vi "DTMF Packet Receiver.vi"() -> ()   [LabVIEW 2011]
uses:
  subVIs_USRP/sub_Chop_Packet.vi
  subVIs_USRP/sub_Ave_Power_And_Thresholding.vi
  subVIs_USRP/sub_Extract_Packet_Boundaries - G.vi
  subVIs_USRP/sub_Extract_Packets.vi
  <instrlib>/niUSRP/niUSRP Fetch Rx Data (CDB Cluster).vi
  subVIs_USRP/subDCOffset.vi
  subVIs_USRP/sub_est_noise_power - G1.vi
  subVIs_DTMF_Student/Proj3_Wireless_DTMF_Receiver.vi
  <vilib>/addons/Modulation/niDMT.lvlib
panel:
  in  "threshold":dbl=97.0
  out "Constellation Graph":T1(graph)
  out "Symbol Rate\n[symbols/sec]":dbl=25000.0 format="%#.6p"
  in  "synchronization parameters":T2={"expected sync location (symbols)"=-1, "sync sequence"=[], "sync location uncertainty (symbols)"=0, "sync indent (symbols)"=0} {"sync sequence" format="%.2f"}
  in  "stop":bool
  in  "Tab Control":T3(tab)=enum."Rx Parameters"
  in  "PN Sequence Order for Sync":i32=31
  in  "Packet Parameters":T4={"Guard Bits "=30, "Sync Bits"=20, "Message Bits"=1024, "Number of Packets \nto Expect"=47}
  out "Received Signal (Raw)":dbl[](graph)
  out "Successfully Received Pkt Num":bool[][](array[boolean])
  out "Packet Reception Percentage (%)":dbl(slide) scale=0.0..100.0
  out "Received Quantized DTMF Signal":dbl[](graph)
  in  "DTMF Settings":T5={"My Phone Number"="", "Ring Tone"=FALSE, "Quantization Level"=4, "\nGray Encoding"=FALSE} {"Quantization Level" items=["2"=2, "4"=4, "8"=8, "16"=16]}
  out "Recovered Message":string
  out "Successfully Received Pkt Num.":bool[][](array[boolean])
  out "Received Digits":string
  in  "Ringtone Path":path=path "C:/Users/Sungeun/Dropbox/Lab/DTMF/VI Source/Project 3/ringtone/Nokia_Original.wav"
  in  "Choose a PSK Format":T6(tab)=enum."QPSK" caption="PSK"
  in  "BPSK System Parameters":T7={"Samples per Symbol"=8, "symbol map"=[], "Differential PSK"=enum."disable", "PSK type"=0} {"PSK type" items=["normal", "shifted", "offset"]; "symbol map" format="%.3f"}
  in  "QPSK System Parameters":T7={"Samples per Symbol"=8, "symbol map"=[], "Differential PSK"=enum."disable", "PSK type"=0} {"PSK type" items=["normal", "shifted", "offset"]; "symbol map" format="%.3f"}
  in  "pi/4 DQPSK System Parameters":T7={"Samples per Symbol"=8, "symbol map"=[], "Differential PSK"=enum."enable", "PSK type"=1} {"PSK type" items=["normal", "shifted", "offset"]; "symbol map" format="%.3f"}
  in  "OQPSK System Parameters":T7={"Samples per Symbol"=8, "symbol map"=[], "Differential PSK"=enum."disable", "PSK type"=2} {"PSK type" items=["normal", "shifted", "offset"]; "symbol map" format="%.3f"}
  in  "8-PSK System Parameters":T7={"Samples per Symbol"=8, "symbol map"=[], "Differential PSK"=enum."disable", "PSK type"=0} {"PSK type" items=["normal", "shifted", "offset"]; "symbol map" format="%.3f"}
  in  "16-PSK System Parameters":T7={"Samples per Symbol"=8, "symbol map"=[], "Differential PSK"=enum."disable", "PSK type"=0} {"PSK type" items=["normal", "shifted", "offset"]; "symbol map" format="%.3f"}
  in  "M":i32=4 min=2 step=2
  in  "Custom System Parameters":T7={"Samples per Symbol"=8, "symbol map"=[], "Differential PSK"=enum."disable", "PSK type"=0} {"PSK type" items=["normal", "shifted", "offset"]; "symbol map" format="%.3f"}
  in  "filter parameters":T8={"Alpha"=0.5, "Filter Length"=6, "TX Filter"=enum."Root Raised Cos"} caption="Matching Filter Parameters" {"Alpha" format="%.2f"}
  in  "Acquisition Duration [sec]":dbl=0.06 format="%#.6p"
  in  "Rx Parameters":T9={"Rx IQ Sampling\nRate [s/sec]"=200000.0, "Rx\nFrequency [Hz]"=915000000.0, "Rx Gain [dB]"=20.0, "Rx Antenna"="RX1"} {"Rx Gain [dB]" format="%#.6p"; "Rx\nFrequency [Hz]" format="%#.6p"; "Rx IQ Sampling\nRate [s/sec]" format="%#.6p"}
  out "Actual Rx Parameters":T9={"Rx IQ Sampling\nRate [s/sec]"=200000.0, "Rx\nFrequency [Hz]"=2500000000.0, "Rx Gain [dB]"=20.0, "Rx Antenna"="RX1"} {"Rx Gain [dB]" format="%#.6p"; "Rx\nFrequency [Hz]" format="%#.6p"; "Rx IQ Sampling\nRate [s/sec]" format="%#.6p"}
  in  "USRP IP Address":refnum<k15>="192.168.10.3"
  out "SNR [dB]":dbl
  out "Sync Found":bool=TRUE
  out "Correct Packets Rx":i16=46
  in  "Continuous Acquire?":bool
  out "Singal & Noise Power":cluster{"signal_power":dbl, "noise_power":dbl}={"signal_power"=0.001168884890875219, "noise_power"=5.163954192250838e-08}
  out "error out":errorcluster
  out "Cumulative Packets Recovered":i16(graph)
  out "Signal and Noise Power Tracking":cluster{"total_power":dbl, "noise_power":dbl}(graph)={"total_power"=0.001168884890875219, "noise_power"=5.163954192250838e-08}
  # "DTMF Packet Receiver"
  # "Guard\nBand"
  # "Sync\nSeq"
  # "Packet\nNumber"
  # "Pad\nData"
  # "Blank\nFrame"
  # "Data"
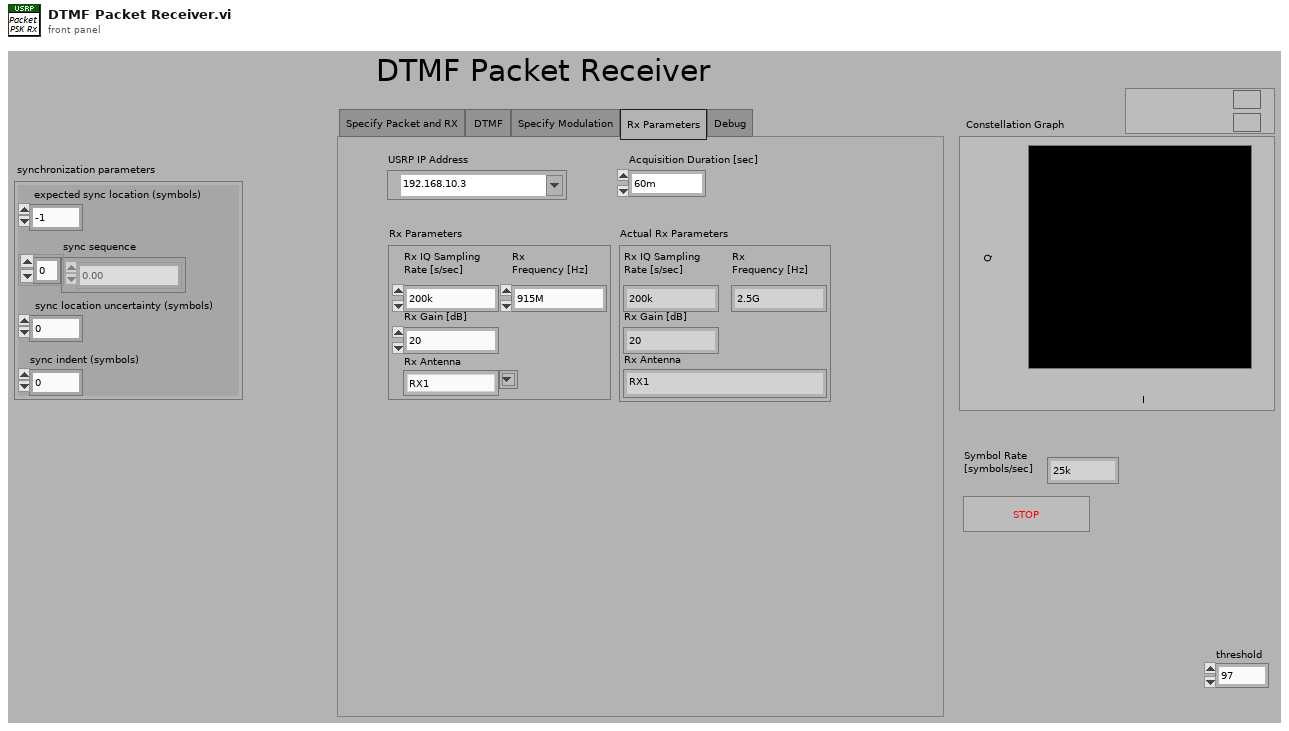
[diagram p1: front panel]
types:
  T1 = cluster{"Decimated Array":dbl[], "Decimated Array":dbl[]}[]
  T2 = cluster{"expected sync location (symbols)":i32, "sync sequence":cdb[], "sync location uncertainty (symbols)":i32, "sync indent (symbols)":i32}
  T3 = enum32{"Specify Packet and RX", "DTMF ", "Specify Modulation", "Rx Parameters", "Debug"}
  T4 = cluster{"Guard Bits ":i32, "Sync Bits":i32, "Message Bits":i32, "Number of Packets \nto Expect":i32}
  T5 = cluster{"My Phone Number":string, "Ring Tone":bool, "Quantization Level":u16, "\nGray Encoding":bool}
  T6 = enum32{"BPSK", "QPSK", "pi/4DQPSK", "OQPSK", "8-PSK", "16-PSK", "Custom"}
  T7 = cluster{"Samples per Symbol":i32, "symbol map":cdb[], "Differential PSK":enum16{"disable", "enable"}, "PSK type":u16}
  T8 = cluster{"Alpha":dbl, "Filter Length":i32, "TX Filter":enum16{"none", "Raised Cosine", "Root Raised Cos", "Gaussian"}}
  T9 = cluster{"Rx IQ Sampling\nRate [s/sec]":dbl, "Rx\nFrequency [Hz]":dbl, "Rx Gain [dB]":dbl, "Rx Antenna":string}
  T10 = cluster{"Packet Array":i32[][], "IP Array of Pkt Nums Received  ":bool[]}
  T11 = cluster{"bit stream ":i8[][], "Sync Valid?":bool[], "Decoded Pkt Numbers":u32[], "Enable?":bool}
  T12 = cluster{"packet_arr":cdb[][], "Packets Valid?":bool}
  T13 = cluster{"PSK type":u16, "Samples per Symbol":i32, "Differential PSK":enum16{"disable", "enable"}, "M":i32}
  T14 = cluster{"PSK system parameters":cluster{"samples per symbol (16)":i32, "symbol map":cdb[], "differential PSK":enum16{"disable", "enable"}, "PSK type":u16}, "pulse shaping filter coefficients":dbl[], "matched filter coefficients":dbl[], "synchronization parameters":cluster{"expected sync location (symbols)":i32, "sync sequence":cdb[], "sync location uncertainty (symbols)":i32, "sync indent (symbols)":i32}, "Sync Bits":i8[]}
  T15 = typedef "niAMT.lvlib/Complex Data Waveform.ctl" = cluster{"t0":dbl, "dt":dbl, "Y":cdb[]}
  T16 = cluster{"constellation":dbl[], "oversampled data":dbl[]}[]
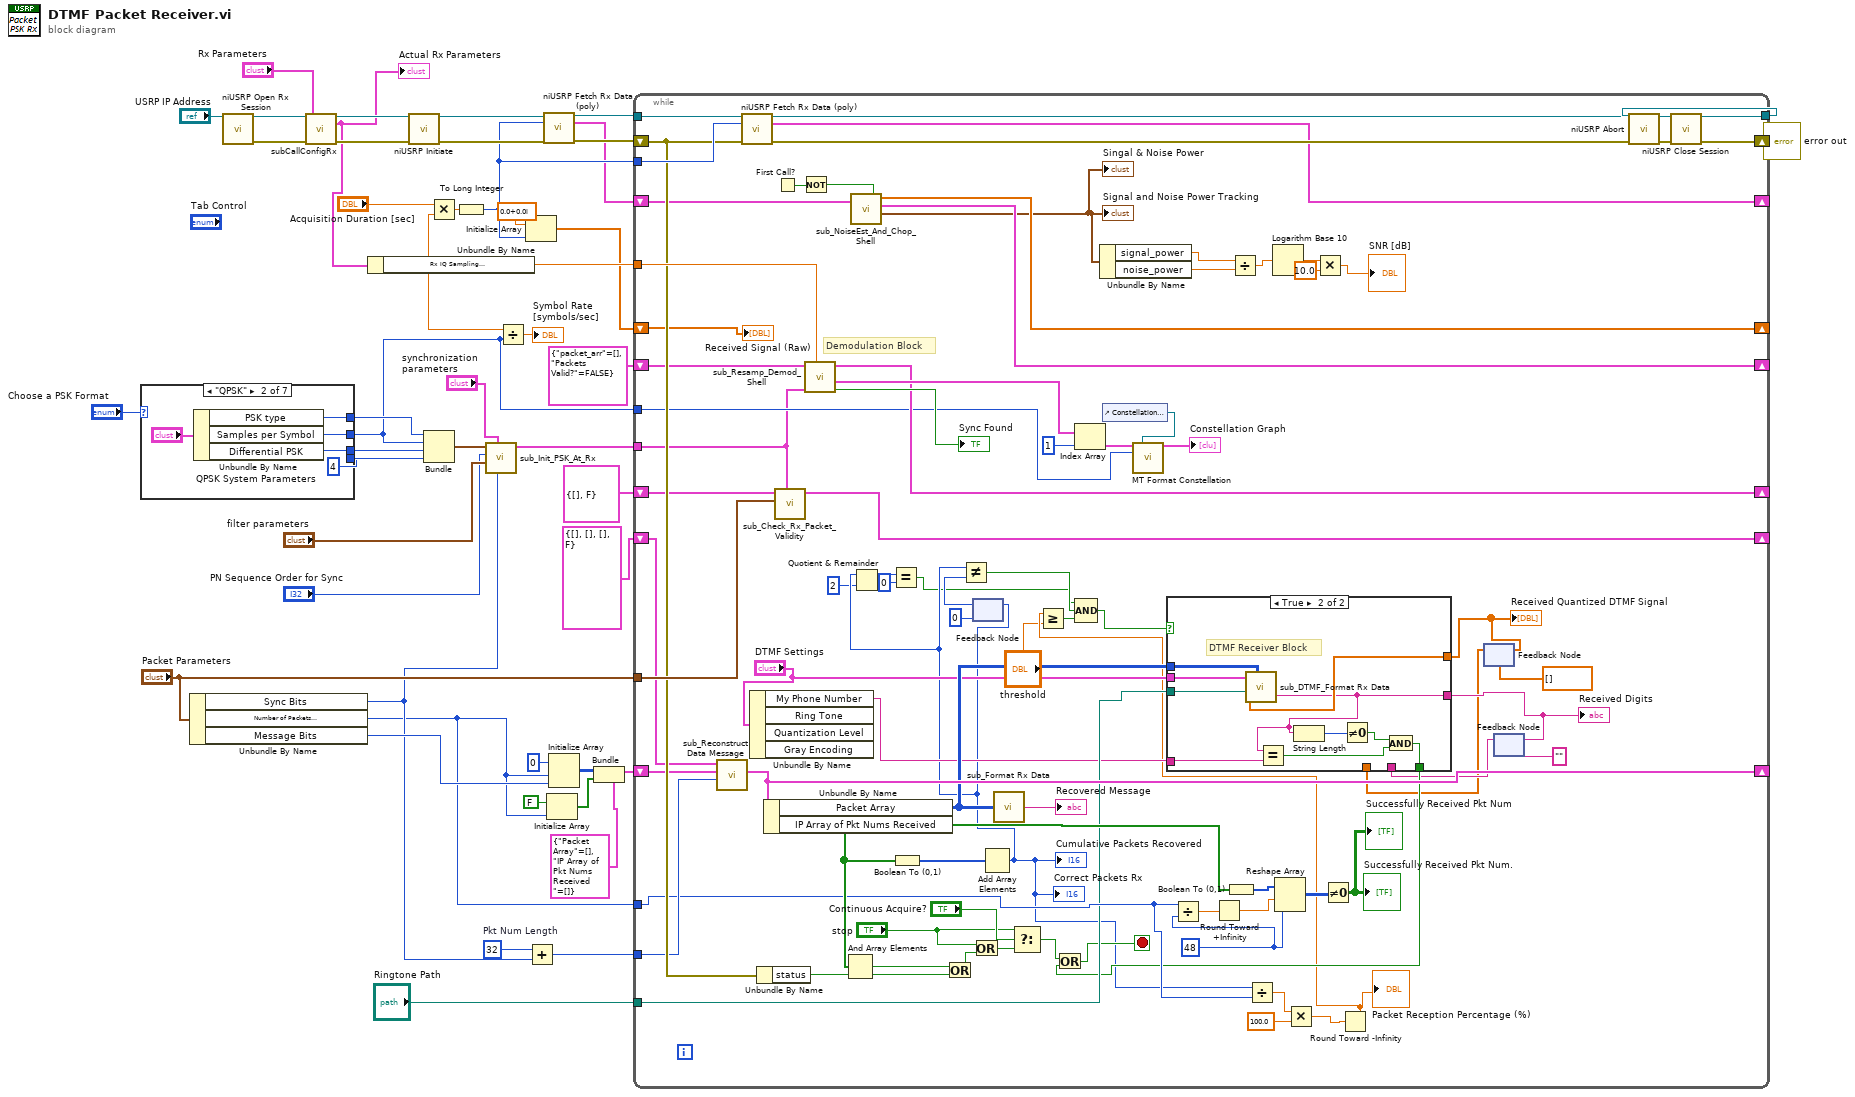
[diagram p0: block diagram]
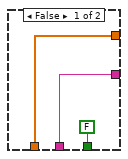
[diagram p2: hidden frame]
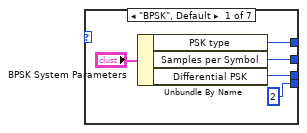
[diagram p3: hidden frame]
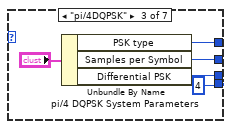
[diagram p4: hidden frame]
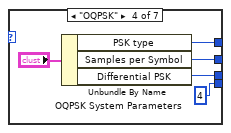
[diagram p5: hidden frame]
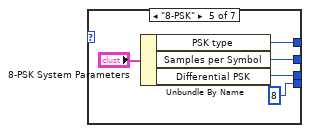
[diagram p6: hidden frame]
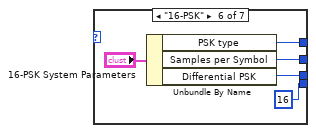
[diagram p7: hidden frame]
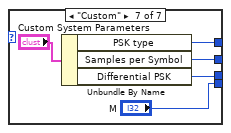
[diagram p8: hidden frame]
diagram:
  w26 = 32  # Pkt Num Length
  n1 = case shown="\"QPSK\"" "Choose a PSK Format" {
    tunnel: [w53 w59 w64 w69 w74 w80 w83] -> w24
    tunnel: [w54 w57 w63 w68 w73 w79 w84] -> w34
    tunnel: [2 ("M-PSK (4)") 4 ("M-PSK (4)") 4 ("M-PSK (4)") 4 ("M-PSK (4)") 8 ("M-PSK (4)") 16 ("M-PSK (4)") "M"] -> w33
    tunnel: [w55 w58 w62 w67 w75 w78 w85] -> w35
    frame "BPSK", Default {
      n2 = Unbundle By Name("BPSK System Parameters") -> ("PSK type"=w55:u16, "Samples per Symbol"=w53:i32, "Differential PSK"=w54:enum16{"disable", "enable"})
    }
    frame "QPSK" {
      n3 = Unbundle By Name("QPSK System Parameters") -> ("PSK type"=w58:u16, "Samples per Symbol"=w59:i32, "Differential PSK"=w57:enum16{"disable", "enable"})
    }
    frame "pi/4DQPSK" {
      n4 = Unbundle By Name("pi/4 DQPSK System Parameters") -> ("PSK type"=w62:u16, "Samples per Symbol"=w64:i32, "Differential PSK"=w63:enum16{"disable", "enable"})
    }
    frame "OQPSK" {
      n5 = Unbundle By Name("OQPSK System Parameters") -> ("PSK type"=w67:u16, "Samples per Symbol"=w69:i32, "Differential PSK"=w68:enum16{"disable", "enable"})
    }
    frame "8-PSK" {
      n6 = Unbundle By Name("8-PSK System Parameters") -> ("PSK type"=w75:u16, "Samples per Symbol"=w74:i32, "Differential PSK"=w73:enum16{"disable", "enable"})
    }
    frame "16-PSK" {
      n7 = Unbundle By Name("16-PSK System Parameters") -> ("PSK type"=w78:u16, "Samples per Symbol"=w80:i32, "Differential PSK"=w79:enum16{"disable", "enable"})
    }
    frame "Custom" {
      n8 = Unbundle By Name("Custom System Parameters") -> ("PSK type"=w85:u16, "Samples per Symbol"=w83:i32, "Differential PSK"=w84:enum16{"disable", "enable"})
    }
  }
  n9 = Unbundle By Name("Packet Parameters") -> ("Sync Bits"=w10:i32, "Number of Packets \nto Expect"=w2:i32, "Message Bits"=w25:i32)
  n10 = call <instrlib>:"niUSRP Open Rx Session.vi"("device names"="USRP IP Address") -> ("session handle out"=w46:refnum<k15>, "error out"=w47:errorcluster)  [unwired: 13 in]
  n11 = call "subCallConfigRx.vi"("session handle"=w46, "Rx Parameters"="Rx Parameters", "error in"=w47) -> ("session handle out"=w44:refnum<k15>, "Actual Rx Parameters"=w27:T9, "error out"=w43:errorcluster)  [unwired: 10 in]
  "Actual Rx Parameters" <- w27
  n12 = Unbundle By Name(w27) -> ("Rx IQ Sampling\nRate [s/sec]"=w21:dbl)
  n13 = call <instrlib>:"niUSRP Initiate.vi"("session handle"=w44, "error in (no error)"=w43) -> ("session handle out"=w6:refnum<k15>, "error out"=w5:errorcluster)  [unwired: 12 in]
  n14 = Bundle("PSK type"=w35, "Samples per Symbol"=w24, "Differential PSK"=w34, "M"=w33) -> (w31:T13)  [unwired: 1 in]
  n15 = Multiply(x="Acquisition Duration [sec]", y=w21) -> (x*y=w49:dbl)
  n16 = To Long Integer(number=w49) -> (32bit integer=w4:i32)
  n17 = call "sub_Init_PSK_At_Rx.vi"("Sync Bits"=w10, "synchronization parameters"="synchronization parameters", "filter parameters"="filter parameters", "PN sequence order (9)"="PN Sequence Order for Sync", "PSK Parameters"=w31) -> ("PSK Init Parameters"=w30:T14)  [unwired: 5 in, 1 out]
  n18 = Divide(x=w21, y=w24) -> (x/y=→"Symbol Rate\n[symbols/sec]":dbl)
  n19 = Initialize Array(cdb 0.0+0.0i ("element"), w4) -> (w12:cdb[])
  n20 = Add(x=w26, y=w10) -> (x+y=w36:i32)
  n21 = call-poly <instrlib>:"niUSRP Fetch Rx Data (poly).vi"("session handle"=w6, "number of samples"=w4, "error in (no error)"=w5) -> ("session handle out"=w8:refnum<k15>, "data"=w3:cluster{"t0":dbl, "dt":dbl, "Y":cdb[]}, "error out"=w7:errorcluster)  [unwired: 9 in, 1 out]
  n22 = Initialize Array(FALSE, w2) -> (w14:bool[])
  n23 = Initialize Array(0, w2, w25) -> (w15:i32[][])
  n24 = Bundle(cluster=T10 {"Packet Array"=[], "IP Array of Pkt Nums Received  "=[]} ("Packet Info"), "Packet Array"=w15, "IP Array of Pkt Nums Received"=w14) -> (w13:T10)
  n25 = while {
    tunnel: w21 -> [w166]
    tunnel: w8 -> [w151]
    tunnel: [w149] -> w40
    tunnel: w4 -> [w148]
    tunnel: "Packet Parameters" -> [w165]
    tunnel: w36 -> [w135]
    tunnel: w30 -> [w131]
    shift-right: [w150] -> w39
    shift-left: w7 -> [w146]
    tunnel: w24 -> [w132]
    shift-right: [w134] -> _
    shift-left: w13 -> [w136]
    shift-right: [w142] -> _
    shift-left: T12 {"packet_arr"=[], "Packets Valid?"=FALSE} -> [w143]
    shift-right: [w138] -> _
    shift-left: cluster{"bit stream":i8[][], "Enable?":bool} {"bit stream"=[], "Enable?"=FALSE} ("Output Bitstream") -> [w141]
    shift-right: [w130] -> _
    shift-left: T11 {"bit stream "=[], "Sync Valid?"=[], "Decoded Pkt Numbers"=[], "Enable?"=FALSE} ("Output Bit Stream") -> [w137]
    shift-right: [w139] -> _
    shift-left: w3 -> [w140]
    shift-right: [w133] -> _
    shift-left: w12 -> [w120]
    tunnel: w2 -> [w121]
    tunnel: "Ringtone Path" -> [w108]
    stop <- w104 stop-if-true
    w124 = 48 ("dimension size")
    # "Demodulation Block"
    n26 = call "sub_Reconstruct Data Message.vi"("Start Loc of Data"=w135, "Packet Info"=w136, "Input Stream"=w137) -> ("Packet Info out"=w134:T10)  [unwired: 8 in]
    n27 = call-poly <instrlib>:"niUSRP Fetch Rx Data (poly).vi"("session handle"=w151, "number of samples"=w148, "error in (no error)"=w146) -> ("session handle out"=w149:refnum<k15>, "data"=w139:cluster{"t0":dbl, "dt":dbl, "Y":cdb[]}, "error out"=w150:errorcluster)  [unwired: 9 in, 1 out]
    n28 = Unbundle By Name("DTMF Settings") -> ("My Phone Number"=w107:string)  [unwired: 3 out]
    n29 = Unbundle By Name(w146) -> ("status"=w145:bool)
    n30 = Unbundle By Name(w134) -> ("Packet Array"=w129:i32[][], "IP Array of Pkt Nums Received"=w128:bool[])
    n31 = First Call?() -> (First Call?: T/F=w153:bool)
    n32 = call "sub_Check_Rx_Packet_Validity.vi"("PSK Init Parameters"=w131, "Packet Parameters"=w165, "Input Bit Stream"=w141) -> ("Output Bit Stream"=w130:T11)  [unwired: 7 in]
    n33 = Not(x=w153) -> (.not. x?=w152:bool)
    n34 = call "sub_Resamp_Demod_Shell.vi"("Rx IQ Sampling\nRate [s/sec]"=w166, "PSK Init Parameters"=w131, "Input Packets"=w143) -> ("Synch Found?"=→"Sync Found":bool, "recovered complex waveform"=w156:T15[], "Output Bitstream"=w138:cluster{"bit stream":i8[][], "Enable?":bool})  [unwired: 3 in]
    n35 = And Array Elements(Boolean array=w128) -> (logical AND=w147:bool)
    n36 = call "sub_NoiseEst_And_Chop_Shell.vi"("data"=w140, "Enable"=w152) -> ("Singal & Noise Power"=w115:cluster{"signal_power":dbl, "noise_power":dbl}, "Output Packets"=w142:cluster{"Packets":cdb[][], "Enable?":bool}, "Delay signal (for plotting use only)"=w133:cdb[])  [unwired: 3 in]
    "Signal and Noise Power Tracking" <- w115
    "Singal & Noise Power" <- w115
    n37 = Boolean To (0,1)(Boolean=w128) -> (0, 1=w164:i16[])
    n38 = Or(x=w147, y=w145) -> (x .or. y?=w144:bool)
    n39 = Or(x="stop", y=w144) -> (x .or. y?=w162:bool)
    n40 = feedback #1(i16 0) -> (w98:i16)
    n41 = Add Array Elements(numeric array=w164) -> (sum=w88:i16)
    "Correct Packets Rx" <- w88
    "Cumulative Packets Recovered" <- w88
    n42 = Quotient & Remainder(x=w88, y=i16 2) -> (x-y*floor(x/y)=w90:i16)  [unwired: 1 out]
    n43 = Equal?(x=w90, y=i16 0) -> (x = y?=w86:bool)
    n44 = Not Equal?(x=w88, y=w98) -> (x != y?=w97:bool)
    n45 = feedback-in #1(w88) -> ()
    n46 = call "sub_Format Rx Data.vi"("Output Packet Array"=w129) -> ("Received Message"=→"Recovered Message":string)
    n47 = Select(t="stop", s="Continuous Acquire?", f=w162) -> (s? t:f=w106:bool)
    n48 = Index Array(array=w156, index=1) -> (element=w155:T15)
    n49 = Unbundle By Name(w115) -> ("signal_power"=w114:dbl, "noise_power"=w113:dbl)
    n50 = control-ref of="Constellation Graph"() -> (w158:refnum<vi>)
    n51 = call <vilib>:"MT Format Constellation.vi"("waveform"=w155, "constellation reference"=w158, "samples per symbol"=w132) -> ("constellation graph"=→"Constellation Graph":T16)  [unwired: 2 in, 10 out]
    n52 = Divide(x=w121, y=w124) -> (x/y=w123:dbl)
    n53 = Round Toward +Infinity(x=w123) -> (ceil(x): smallest int >= x=w122:dbl)
    n54 = Boolean To (0,1)(Boolean=w128) -> (0, 1=w127:i16[])
    n55 = Divide(x=w114, y=w113) -> (x/y=w112:dbl)
    n56 = Divide(x=w88, y=w121) -> (x/y=w117:dbl)
    n57 = Logarithm Base 10(1:w112) -> (0:w111:dbl)
    n58 = Reshape Array(w127, w122, w124) -> (w126:i16[][])
    n59 = Multiply(x=w117, y=100.0) -> (x*y=w116:dbl)
    n60 = Multiply(x=w111, y=10.0) -> (x*y=→"SNR [dB]":dbl)
    n61 = Not Equal To 0?(x=w126) -> (x != 0?=→"Successfully Received Pkt Num." →"Successfully Received Pkt Num":bool[][])
    n62 = Round Toward -Infinity(1:w116) -> (0:w103:dbl)
    "Packet Reception Percentage (%)" <- w103
    n63 = Greater Or Equal?(x=w103, y="threshold") -> (x >= y?=w101:bool)
    n64 = Compound Arithmetic op=AND(w86, w97, w101) -> (w100:bool)
    n65 = feedback #2(dbl[] [] ("dequants")) -> (w93:dbl[])
    n66 = feedback #3("" ("Received Digits")) -> (w95:string)
    n67 = case shown="True" w100 {
      tunnel: w129 -> [_ w179]
      tunnel: "DTMF Settings" -> [_ w178]
      tunnel: [w167 w177] -> w94
      tunnel: w108 -> [_ w176]
      tunnel: [w168 w172] -> w96
      tunnel: w107 -> [_ w171]
      tunnel: [FALSE w170] -> w105
      tunnel: w95 -> [w168 _]
      tunnel: w93 -> [w167 _]
      frame False {
      }
      frame True {
        # "DTMF Receiver Block"
        n68 = call "sub_DTMF_Format Rx Data.vi"("DTMF Settings"=w178, "Ringtone Path"=w176, "Output Packet Array"=w179) -> ("dequants"=w177:dbl[], "Received Digits"=w172:string)  [unwired: 1 in, 1 out]
        n69 = Equal?(x=w172, y=w171) -> (x = y?=w173:bool)
        n70 = String Length(string=w172) -> (length=w175:i32)
        n71 = Not Equal To 0?(x=w175) -> (x != 0?=w174:bool)
        n72 = And(x=w174, y=w173) -> (x .and. y?=w170:bool)
      }
    }
    "Received Quantized DTMF Signal" <- w94
    "Received Digits" <- w96
    n73 = Or(x=w106, y=w105) -> (x .or. y?=w104:bool)
    n74 = feedback-in #2(w94) -> ()
    n75 = feedback-in #3(w96) -> ()
    "Received Signal (Raw)" <- w120
  }
  n76 = call <instrlib>:"niUSRP Abort.vi"("session handle"=w40, "error in (no error)"=w39) -> ("session handle out"=w41:refnum<k15>, "error out"=w42:errorcluster)  [unwired: 12 in]
  n77 = call <instrlib>:"niUSRP Close Session.vi"("session handle"=w41, "error in (no error)"=w42) -> ("error out"=→"error out":errorcluster)  [unwired: 13 in]
